vi "rtest.vi"() -> ()   [LabVIEW 2015]
panel:
  in  "Activate?":bool
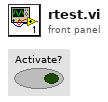
[diagram p1: front panel]
types:
  T1 = enum32{"Invalid", "Standard", "Closed", "Hidden", "Minimized", "Maximized"}
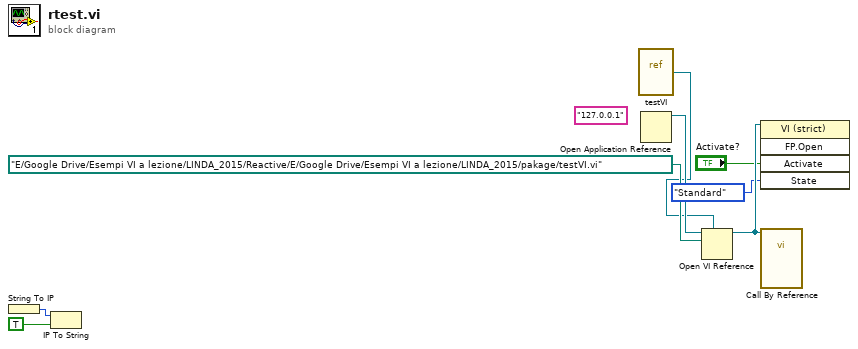
[diagram p0: block diagram]
diagram:
  (unwired) "127.0.0.1" ("machine name (\"\":  open local reference)")
  n1 = String To IP() -> (0:w1:u32)  [unwired: 1 in]
  n2 = IP To String(1:TRUE ("dot notation? (F)"), 2:w1) -> ()  [unwired: 1 out]
  n3 = vi-ref "testVI.vi"() -> (w6:refnum<vi>)
  n4 = Open Application Reference() -> (3:w8:refnum<vi>)  [unwired: 4 in, 1 out]
  n5 = Open VI Reference(type specifier VI Refnum (for type only)=w6, application reference (local)=w8, vi path=path "E:/Google Drive/Esempi VI a lezione/LINDA_2015/Reactive/E/Google Drive/Esempi VI a lezione/LINDA_2015/pakage/testVI.vi") -> (vi reference=w5:refnum<vi>)  [unwired: 3 in, 1 out]
  n6 = invoke class="VI (strict)" method="FP.Open"(reference=w5, "Activate"="Activate?", "State"=T1."Standard") -> ()  [unwired: 2 in, 5 out]
  n7 = call-by-ref "?"(reference=w5) -> ()  [unwired: 13 in, 2 out]
